vi "Convert RGB Cluster to RGB String.vi"(8 "error in (no error)":errorcluster, 10 "RGB":cluster{"R":i32, "G":i32, "B":i32}, 11 "Initial String":string) -> (0 "error out":errorcluster, 2 "RGB String":string)   [LabVIEW 2020, in "Yokogawa GX Series.lvlib"]
doc: "Converts RGB cluster to string and concatenates to initial string."
uses:
  <instrlib>/Yokogawa GX Series/Yokogawa GX Series.lvlib
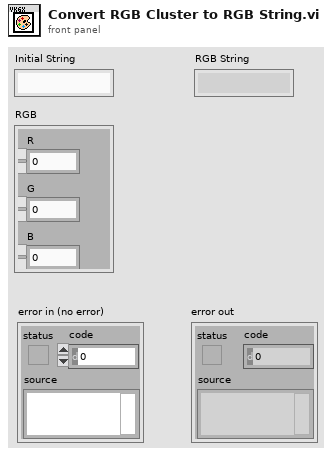
[diagram p1: front panel]
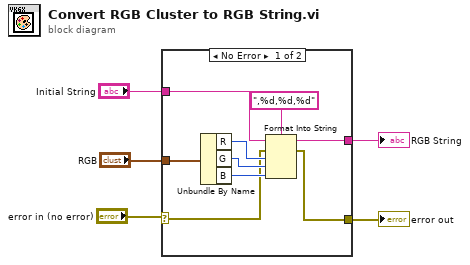
[diagram p0: block diagram]
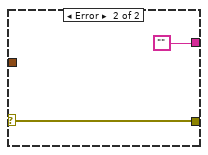
[diagram p2: hidden frame]
diagram:
  n1 = case shown="No Error" "error in (no error)" {
    selector: "error in (no error)" -> [w6 w16]
    tunnel: "RGB" -> [w14 _]
    tunnel: [w10 ""] -> w4
    tunnel: [w9 w16] -> w3
    tunnel: "Initial String" -> [w7 _]
    frame No Error {
      n2 = Unbundle By Name(w14) -> ("R"=w13:i32, "G"=w12:i32, "B"=w11:i32)
      n3 = Format Into String(format string=",%d,%d,%d", initial string=w7, error in=w6, w13, w12, w11) -> (resulting string=w10:string, error out=w9:errorcluster)
    }
    frame Error {
    }
  }
  "RGB String" <- w4
  "error out" <- w3
